vi "Init.vi"() -> (0 "Error out":errorcluster, 3 "Base Actor out":refnum<class "Base Actor.lvclass">)   [LabVIEW 2020, in "jettl.lvlib" / "Actor.lvlib" / "Base Actor.lvclass"]
uses:
  Base Actor.lvclass
  Actor.lvlib
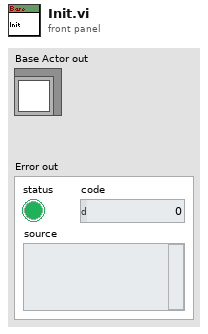
[diagram p1: front panel]
types:
  T1 = typedef "jettl.lvlib/Actor.lvlib/Msg Set.ctl" = set{refnum<class "Msg.lvclass">}
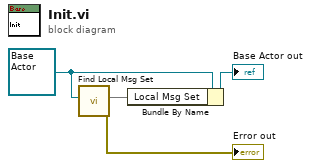
[diagram p0: block diagram]
diagram:
  w2 = refnum<class "Base Actor.lvclass"> refnum ("jettl Event Actor out")
  n1 = call "Find Local Msg Set.vi"("Variant (X Actor.lvclass)"=w2) -> ("Error out"=→"Error out":errorcluster, "Local Msg Set"=w3:T1)  [unwired: 9 in]
  n2 = Bundle By Name(cluster=w2, "Local Msg Set"=w3) -> (→"Base Actor out":refnum<class "Base Actor.lvclass">)
